vi "Apply Wheel State.vi"(8 "error in (no error)":errorcluster, 10 "wheel state in":T1, 11 "steering wheel in":refnum<class "NI_Robotics_Steering Wheel.lvclass">) -> (0 "error out":errorcluster, 2 "wheel state out":T1, 3 "steering wheel out":refnum<class "NI_Robotics_Steering Wheel.lvclass">)   [LabVIEW 2017, in "NI_Robotics_Steering Wheel.lvclass"]
uses:
  <vilib>/robotics/Steering/Steering Wheel/NI_Robotics_Steering Wheel.lvclass
  c:/Program Files (x86)/National Instruments/LabVIEW 2017/vi.lib/robotics/Steering/Wheel/NI_Robotics_Wheel.lvclass
  <vilib>/robotics/Steering/Wheel/Wheel State.ctl
  <vilib>/robotics/Steering/Steering Wheel/NI_Robotics_Steering Wheel.lvclass/NI_Robotics_Steering Wheel.ctl
  <vilib>/robotics/Steering/Wheel/NI_Robotics_Wheel.lvclass/NI_Robotics_Wheel.ctl
  <vilib>/robotics/Actuation/Motor Communication/Update Motor Angle Setpoint.vi
  <vilib>/robotics/Actuation/Motor Communication/Update Motor Velocity Setpoint.vi
  <vilib>/robotics/Actuation/Motor Communication/Check if Valid.vi
  <vilib>/robotics/Utilities/Generate Error.vi
  <vilib>/robotics/Actuation/Motor Communication/NI_Robotics_Motor Communication.lvclass
  <vilib>/robotics/Steering/Wheel/NI_Robotics_Wheel.lvclass
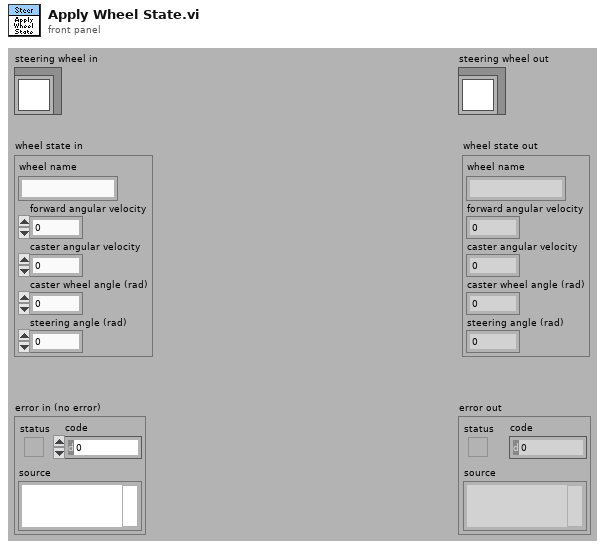
[diagram p1: front panel]
types:
  T1 = typedef "NI_Robotics_Wheel.lvclass/Wheel State.ctl" = cluster{"wheel name":string, "forward angular velocity":dbl, "caster angular velocity":dbl, "caster wheel angle (rad)":dbl, "steering angle (rad)":dbl}
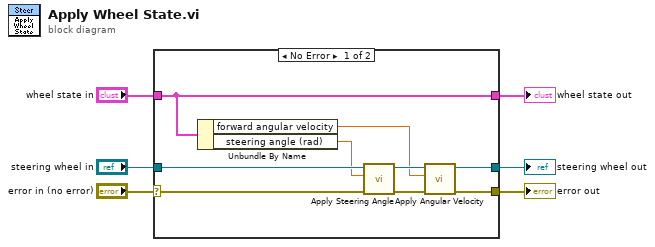
[diagram p0: block diagram]
diagram:
  n1 = case shown="No Error" "error in (no error)" {
    selector: "error in (no error)" -> [w13 w17]
    tunnel: "steering wheel in" -> [w14 w18]
    tunnel: [w8 w18] -> w4
    tunnel: [w9 w17] -> w3
    tunnel: "wheel state in" -> [w15 w16]
    tunnel: [w15 w16] -> w1
    frame No Error {
      n2 = Unbundle By Name(w15) -> ("forward angular velocity"=w10:dbl, "steering angle (rad)"=w7:dbl)
      n3 = call <vilib>:"Apply Steering Angle.vi"("error in (no error)"=w13, "steering angle (rad)"=w7, "steering wheel in"=w14) -> ("error out"=w11:errorcluster, "steering wheel out"=w12:refnum<class "NI_Robotics_Steering Wheel.lvclass">)  [unwired: 7 in]
      n4 = call <vilib>:"Apply Angular Velocity.vi"("error in (no error)"=w11, "forward angular velocity"=w10, "wheel in"=w12) -> ("error out"=w9:errorcluster, "wheel out"=w8:refnum<class "NI_Robotics_Steering Wheel.lvclass">)  [unwired: 7 in]
    }
    frame Error {
    }
  }
  "error out" <- w3
  "steering wheel out" <- w4
  "wheel state out" <- w1
